vi "20211015_00.vi"() -> ()   [LabVIEW 2019]
panel:
  out "sum":dbl
  in  "Nums array":dbl[](array[numeric])
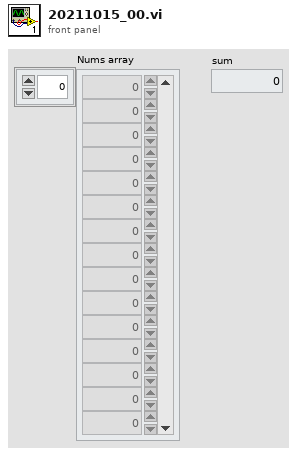
[diagram p1: front panel]
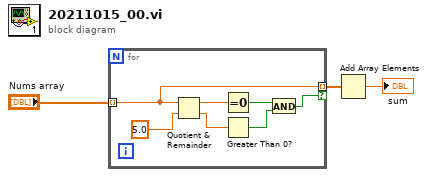
[diagram p0: block diagram]
diagram:
  n1 = for {
    tunnel: "Nums array" -> [w5] mode=indexing
    tunnel: [w5] -> w2 mode=indexing if=w4
    n2 = Quotient & Remainder(x=w5, y=5.0) -> (x-y*floor(x/y)=w9:dbl, floor(x/y)=w8:dbl)
    n3 = Equal To 0?(x=w9) -> (x = 0?=w7:bool)
    n4 = Greater Than 0?(x=w8) -> (x > 0?=w6:bool)
    n5 = And(x=w7, y=w6) -> (x .and. y?=w4:bool)
  }
  n6 = Add Array Elements(numeric array=w2) -> (sum=→"sum":dbl)
